vi "ProcessRS232Updates.vi"(11 "MockDisplaceSettings":T1={"BufferUpdateFIFO"="MockDisplaceCommand", "DisplaceMeasurementMemory"="MockDisplaceMeasurements"}) -> ()   [LabVIEW 2016, in "FPGAMockDisplace.lvlib"]
uses:
  FPGAMockDisplace.lvlib
  DataTypes/MockDisplaceSettings.ctl
  <vilib>/rvi/Emulation/niFpgaGetClockAttributes.vi
  <vilib>/rvi/Emulation/niFpgaSctlEmulationGetInTimedLoop.vi
  <vilib>/rvi/Emulation/niFpgaEmulationReportErrorSimple.vi
  <vilib>/rvi/eio/common/nirviEmuTemplateMethod_errors.vi
  <vilib>/rvi/DataTransferAndStorage/Container/Common/niFpgaContainerExecOnDevCompGetState.vi
  <vilib>/rvi/Emulation/niFpgaEmulationIsFPGAContextNoSignature.vi
  <vilib>/rvi/DataTransferAndStorage/Container/Common/niFpgaContainerGetUniqueNameForEmu.vi
  <vilib>/rvi/Emulation/niFpgaProcessEmulError.vi
  <vilib>/rvi/errors/nirviReportUnexpectedCaseInternalError (U32).vi
  <vilib>/rvi/Memory/Memory_Emulation/niFpgaMemoryEmulationCacheClearOnFirstRun.vi
  <vilib>/rvi/Memory/Memory_Emulation/nirvimemoryEmulationManagerCache_MakeExclusive.vi
  <vilib>/rvi/Memory/Memory_Emulation/niFpgaMemoryEmulationValidateCache.vi
  <vilib>/rvi/Memory/Memory_Emulation/nirvimemoryEmulationManagerCache_InsertValue.vi
  <vilib>/Utility/error.llb/Clear Errors.vi
  <vilib>/rvi/Memory/Memory_Emulation/nirvimemoryEmulationManagerCache_ReleaseExclusive.vi
  <vilib>/rvi/Memory/Memory_Emulation/nirvimemoryEmulationManagerCache_GetValue.vi
  <vilib>/rvi/Memory/Memory_Emulation/nirvimemoryEmulationManagerCache_SetValue.vi
  <vilib>/rvi/Emulation/niFpgaSctlEmulationResourceMgr.vi
  <vilib>/rvi/Emulation/niFpgaCriticalErrorInLSC.vi
  <vilib>/eio/EIOMethodNode/EIOMethodNode.xnode
  <vilib>/rvi/DataTransferAndStorage/Container/XNode/niFpgaContainer.xnode
  <vilib>/rvi/Memory/Memory_Emulation/niFpgaMemoryEmulationRefIn.vi
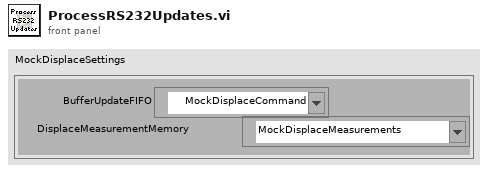
[diagram p1: front panel]
types:
  T1 = typedef "FPGAMockDisplace.lvlib/MockDisplaceSettings.ctl" = cluster{"BufferUpdateFIFO":refnum<k21>, "DisplaceMeasurementMemory":refnum<k21>}
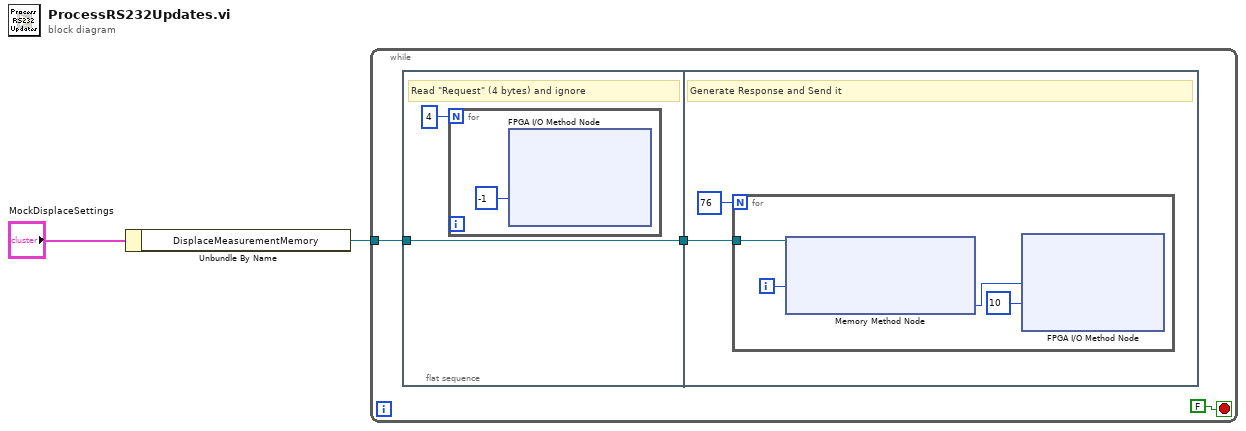
[diagram p0: block diagram]
diagram:
  n1 = Unbundle By Name("MockDisplaceSettings") -> ("DisplaceMeasurementMemory"=w2:refnum<k21>)
  n2 = while {
    tunnel: w2 -> [w4]
    stop <- FALSE stop-if-true
    n3 = flat-sequence {
      tunnel: [w6] -> w5
      tunnel: w4 -> [w6]
      tunnel: w5 -> [w10]
      frame #0 {
        # "Read \"Request\" (4 bytes) and ignore"
        n4 = for {
          N: 4 -> [_]
          n5 = xnode "FPGA I/O Method Node"("Timeout (ms)"=-1) -> ()  [unwired: 1 in, 3 out]
        }
      }
      frame #1 {
        # "Generate Response and Send it"
        n6 = for {
          N: 76 -> [_]
          tunnel: w10 -> [w14]
          i -> [w11]
          n7 = xnode ("Memory Method Node")("Address"=w11, "Memory In"=w14) -> ("Data"=w13:u8)  [unwired: 1 out]
          n8 = xnode "FPGA I/O Method Node"("Data"=w13, "Timeout (ms)"=10) -> ()  [unwired: 1 in, 2 out]
        }
      }
    }
  }
